vi "Run.vi"(8 "error in (no error)":errorcluster, 9 "Time Ratio used":dbl, 10 "Maze (0: Empty, -1: Enemy. >0: Teammate":i32[][](array[numeric]), 11 "Snail In":refnum<class "Cautious Random Location.lvclass">) -> (0 "error out":errorcluster, 1 "Direction":T1, 2 "Action":T2, 3 "Snail Out":refnum<class "Cautious Random Location.lvclass">, 4 "Replicated":refnum<class "Square.lvclass">)   [LabVIEW 2015, in "Cautious Random Location.lvclass"]
uses:
  Cautious Random Location.lvclass
  Type Defs/Action Enum.ctl
  Type Defs/Direction Enum.ctl
  Square/Square.lvclass
  Cautious Random Location.lvclass/Cautious Random Location.ctl
  Common/Reverse Direction.vi
  SubVIs/Read-Only Globals.vi
  Type Defs/SB Type Defs.lvlib
  Common/Common.lvlib
panel:
  # "NOTICE - YOU MUST NOT REMOVE THIS NOTICE. PER THE FOLLOWING LICENSE, YOU MAY REPRODUCE THIS SOFTWARE PROVIDED YOU FOLLOW THE TERMS\nOF THE LICENSE.\n\n---BEGIN BSD LICENSE (http://opensource.org/licenses/BSD-2-Clause)---\nCopyright (c) 2015, Endigit, Inc. <robert@endigit.com>\nAll rights reserved.\n\nRedistribution and use in source and binary forms, with or without modification, are permitted provided that the following conditions are met:\n\n1. Redistributions of source code must retain the above copyright notice, this list of conditions and the following disclaimer.\n\n2. Redistributions in binary form must reproduce the above copyright notice, this list of conditions and the following disclaimer in the documentation and/or other \nmaterials provided with the distribution.\n\nTHIS SOFTWARE IS PROVIDED BY THE COPYRIGHT HOLDERS AND CONTRIBUTORS \"AS IS\" AND ANY EXPRESS OR IMPLIED WARRANTIES, INCLUDING, BUT NOT \nLIMITED TO, THE IMPLIED WARRANTIES OF MERCHANTABILITY AND FITNESS FOR A PARTICULAR PURPOSE ARE DISCLAIMED. IN NO EVENT SHALL THE COPYRIGHT \nHOLDER OR CONTRIBUTORS BE LIABLE FOR ANY DIRECT, INDIRECT, INCIDENTAL, SPECIAL, EXEMPLARY, OR CONSEQUENTIAL DAMAGES (INCLUDING, BUT NOT \nLIMITED TO, PROCUREMENT OF SUBSTITUTE GOODS OR SERVICES; LOSS OF USE, DATA, OR PROFITS; OR BUSINESS INTERRUPTION) HOWEVER CAUSED AND ON \nANY THEORY OF LIABILITY, WHETHER IN CONTRACT, STRICT LIABILITY, OR TORT (INCLUDING NEGLIGENCE OR OTHERWISE) ARISING IN ANY WAY OUT OF THE USE \nOF THIS SOFTWARE, EVEN IF ADVISED OF THE POSSIBILITY OF SUCH DAMAGE.\n---END BSD LICENSE---"
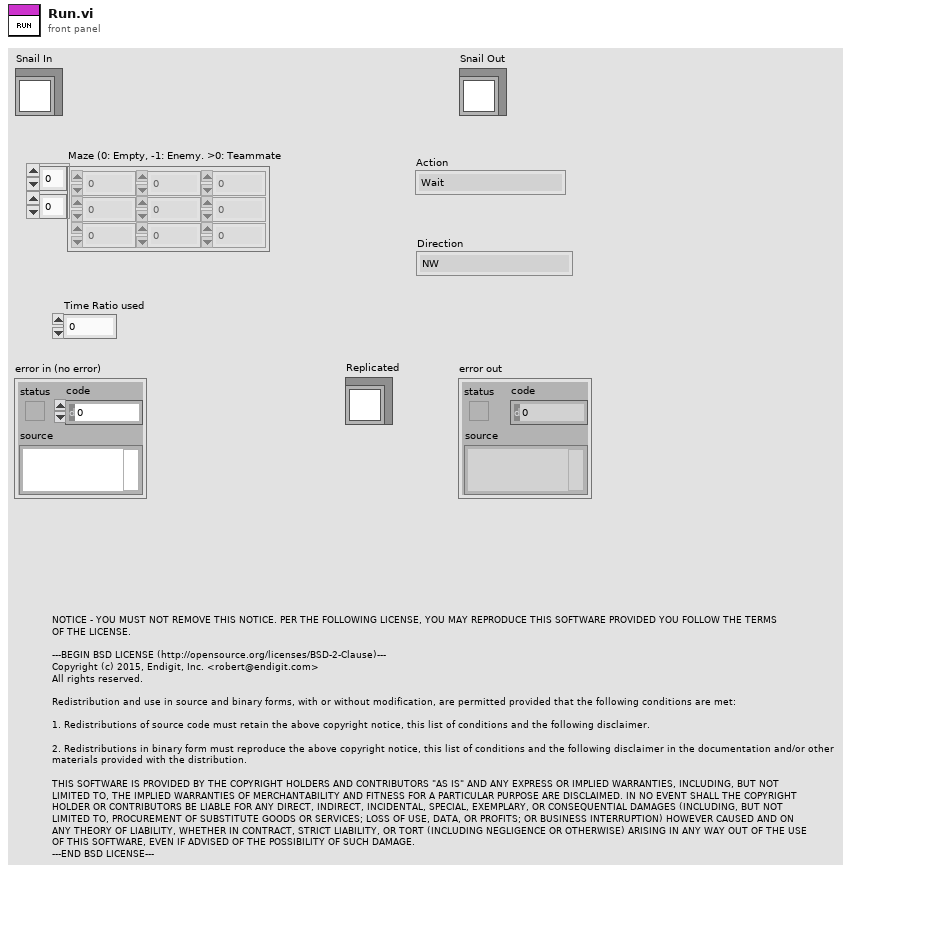
[diagram p1: front panel]
types:
  T1 = typedef "SB Type Defs.lvlib/Direction Enum.ctl" = enum16{"NW", "N", "NE", "E", "SE", "S", "SW", "W"}
  T2 = typedef "SB Type Defs.lvlib/Action Enum.ctl" = enum16{"Wait", "Move", "Attack", "Replicate"}
  T3 = typedef "Common.lvlib/Position.ctl" = cluster{"Column":i32, "Row":i32}
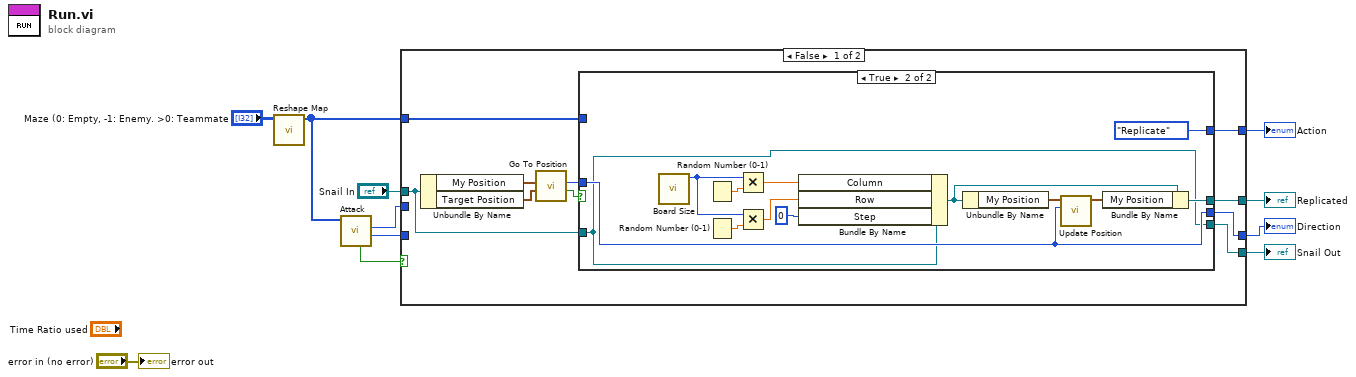
[diagram p0: block diagram]
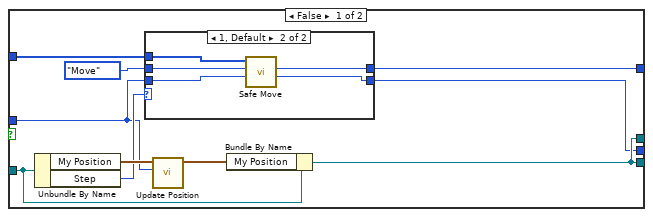
[diagram p2: hidden frame]
diagram:
  n1 = call "Reshape Map.vi"("Maze (0: Empty, -1: Enemy. >0: Teammate"="Maze (0: Empty, -1: Enemy. >0: Teammate") -> ("Map"=w1:i32[])  [unwired: 9 in, 1 out]
  n2 = call "Attack.vi"("Maze (0: Empty, -1: Enemy. >0: Teammate"=w1) -> ("Direction"=w3:i32, "Action"=w4:T2, "Enemy Found?"=w5:bool)  [unwired: 5 in, 3 out]
  n3 = case shown="False" w5 {
    tunnel: [w12 w54] -> w9
    tunnel: "Snail In" -> [w19 w52]
    tunnel: [w15 w52] -> w7
    tunnel: [w13 w53] -> w6
    tunnel: w4 -> [_ w54]
    tunnel: w3 -> [_ w53]
    tunnel: [w16 w52] -> w2
    tunnel: w1 -> [w14 _]
    frame False {
      n4 = Unbundle By Name(w19) -> ("My Position"=w21:cluster{"Column":i32, "Row":i32}, "Target Position"=w20:cluster{"Column":i32, "Row":i32})
      n5 = call "Go To Position.vi"("Target Position"=w20, "My Position"=w21) -> ("Arrived?"=w18:bool, "Direction"=w17:T1)  [unwired: 7 in, 1 out]
      n6 = case shown="True" w18 {
        tunnel: [w25 Action_Enum."Replicate" ("x")] -> w12
        tunnel: w19 -> [w30 w40]
        tunnel: [w28 w40] -> w16
        tunnel: w17 -> [w23 w42]
        tunnel: [w22 w42] -> w13
        tunnel: [w28 w41] -> w15
        tunnel: w14 -> [w26 _]
        frame False {
          n7 = Unbundle By Name(w30) -> ("My Position"=w31:cluster{"Column":i32, "Row":i32}, "Step"=w27:i32)
          n8 = case shown="1, Default" w27 {
            tunnel: w26 -> [_ w38]
            tunnel: w23 -> [w32 w37]
            tunnel: [w33 w35] -> w25
            tunnel: Action_Enum."Move" ("f") -> [w33 w36]
            tunnel: [w32 w34] -> w22
            frame 0 {
            }
            frame 1, Default {
              n9 = call "Safe Move.vi"("Direction in"=w37, "Action in"=w36, "Map"=w38) -> ("Direction"=w34:T1, "Action"=w35:T2)  [unwired: 7 in]
            }
          }
          n10 = call "Update Position.vi"("Direction"=w23, "Position in"=w31) -> ("Position out"=w29:T3)  [unwired: 9 in]
          n11 = Bundle By Name(cluster=w30, "My Position"=w29) -> (w28:refnum<class "Cautious Random Location.lvclass">)
        }
        frame True {
          n12 = call "Board Size.vi"() -> ("Board Size"=w49:i32)  [unwired: 11 in]
          n13 = Random Number (0-1)() -> (number: 0 to 1=w48:dbl)
          n14 = Random Number (0-1)() -> (number: 0 to 1=w50:dbl)
          n15 = Multiply(x=w49, y=w48) -> (x*y=w47:dbl)
          n16 = Multiply(x=w49, y=w50) -> (x*y=w46:dbl)
          n17 = Bundle By Name(cluster=w40, "Column"=w47, "Row"=w46, "Step"=0) -> (w45:refnum<class "Cautious Random Location.lvclass">)
          n18 = Unbundle By Name(w45) -> ("My Position"=w44:cluster{"Column":i32, "Row":i32})
          n19 = call "Update Position.vi"("Direction"=w42, "Position in"=w44) -> ("Position out"=w43:T3)  [unwired: 9 in]
          n20 = Bundle By Name(cluster=w45, "My Position"=w43) -> (w41:refnum<class "Cautious Random Location.lvclass">)
        }
      }
    }
    frame True {
    }
  }
  "Snail Out" <- w2
  "Action" <- w9
  "Replicated" <- w7
  "Direction" <- w6
  "error out" <- "error in (no error)"
